vi "PI_GCS2_Sample_Application_2_Controllers.vi"() -> ()   [LabVIEW 2020]
doc: "This VI demonstrates how to initialize two PI GCS2 systems and how to query the help answers. \nThe diagram shows how to combine the driver VIs for these tasks. \n\nWarning: Before running this VI, modify the interface settings on the block diagram to reflect your configuration. The predefined settings provided with the VI probably do not match your system."
uses:
  Interface Settings.ctl
panel:
  out "Help string Sys. 2":string
  out "Identification Sys. 2":string
  out "Connected Axis System 2":string[](array[string])
  out "Help string Sys. 1":string
  in  "stop":bool
  in  "error in":errorcluster
  out "Running":bool caption="Configuration_Setup.vis running"
  out "error out":errorcluster
  out "Connected Axis System 1":string[](array[string])
  out "Identification Sys. 1":string
  # "This VI demonstrates how to initialize two PI GCS2 systems and how to query their help answer. \nThe diagram shows how to combine the driver VIs for these tasks. \n\nWarning: Before running this VI, modify the interface settings on the block diagram to reflect your configuration. The predefined \n                 settings provided with the VI probably do not match your system."
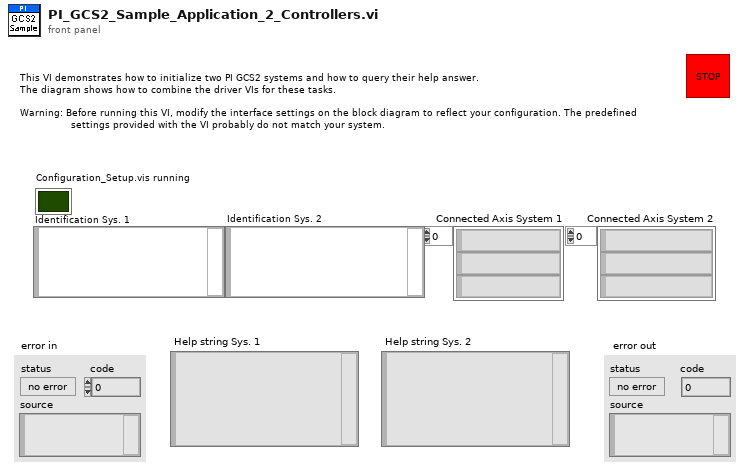
[diagram p1: front panel]
types:
  T1 = typedef "Interface Settings.ctl" = cluster{"Interface":u16, "Timeout":u32, "RS232 settings":cluster{"Portnumber":u8, "Baudrate":u16}, "TCP/IP settings":cluster{"Host address/name":string, "Port":i32, "Board":i32, "TCP/IP Search?":bool}, "USB settings":cluster{"S/N":string, "USB Search?":bool}, "DaisyChain settings":cluster{"Register DC":bool, "DaisyChain Search?":bool, "Device ID":i32}, "DLL for Device":u16}
  T2 = enum16{"Do not reference", "Reference switch", "Negative limit switch", "Positive limit switch"}[]
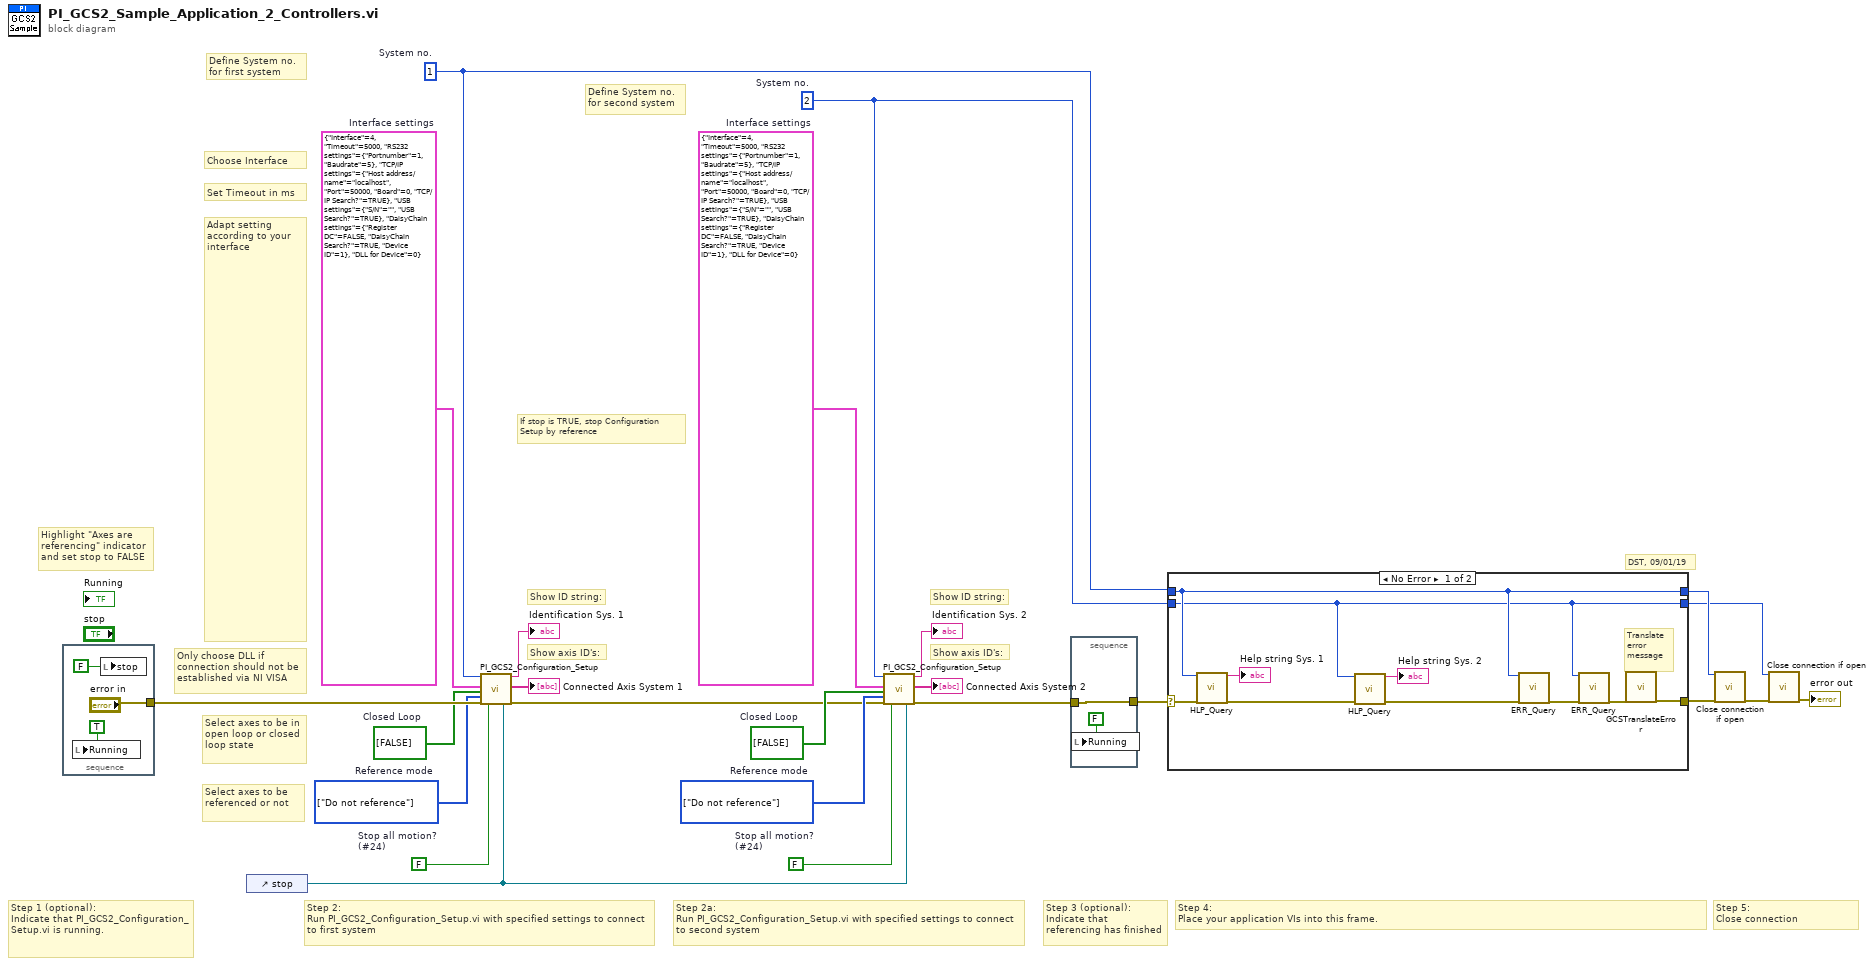
[diagram p0: block diagram]
diagram:
  w5 = T1 {"Interface"=4, "Timeout"=5000, "RS232 settings"={"Portnumber"=1, "Baudrate"=5}, "TCP/IP settings"={"Host address/name"="localhost", "Port"=50000, "Board"=0, "TCP/IP Search?"=TRUE}, "USB settings"={"S/N"="", "USB Search?"=TRUE}, "DaisyChain settings"={"Register DC"=FALSE, "DaisyChain Search?"=TRUE, "Device ID"=1}, "DLL for Device"=0}  # Interface settings
  w6 = T1 {"Interface"=4, "Timeout"=5000, "RS232 settings"={"Portnumber"=1, "Baudrate"=5}, "TCP/IP settings"={"Host address/name"="localhost", "Port"=50000, "Board"=0, "TCP/IP Search?"=TRUE}, "USB settings"={"S/N"="", "USB Search?"=TRUE}, "DaisyChain settings"={"Register DC"=FALSE, "DaisyChain Search?"=TRUE, "Device ID"=1}, "DLL for Device"=0}  # Interface settings
  w16 = FALSE  # Stop all motion? (#24)
  w15 = T2 [enum."Do not reference"] items=["Do not reference", "Reference switch", "Negative limit switch", "Positive limit switch"]  # Reference mode
  w14 = bool[] [FALSE]  # Closed Loop
  w4 = 2  # System no.
  w17 = FALSE  # Stop all motion? (#24)
  w18 = T2 [enum."Do not reference"] items=["Do not reference", "Reference switch", "Negative limit switch", "Positive limit switch"]  # Reference mode
  w19 = bool[] [FALSE]  # Closed Loop
  w2 = 1  # System no.
  # "Step 2a: \nRun PI_GCS2_Configuration_Setup.vi with specified settings to connect to second system"
  # "Define System no. for second system"
  # "Show axis ID's:"
  # "Show ID string:"
  # "Step 5: \nClose connection"
  # "Define System no.\nfor first system"
  # "Select axes to be referenced or not"
  # "Select axes to be in open loop or closed loop state"
  # "Adapt setting according to your interface"
  # "Set Timeout in ms"
  # "Choose Interface"
  # "Only choose DLL if connection should not be established via NI VISA"
  # "If stop is TRUE, stop Configuration\nSetup by reference"
  # "Step 4: \nPlace your application VIs into this frame."
  # "DST, 09/01/19"
  # "Step 3 (optional): \nIndicate that referencing has finished"
  # "Step 2: \nRun PI_GCS2_Configuration_Setup.vi with specified settings to connect to first system"
  # "Step 1 (optional): \nIndicate that PI_GCS2_Configuration_Setup.vi is running."
  # "Highlight \"Axes are\nreferencing\" indicator\nand set stop to FALSE"
  # "Show axis ID's:"
  # "Show ID string:"
  n1 = stacked-sequence {
    tunnel: ["error in"] -> w23
    frame #0 {
      n2 = local write "Running"(TRUE ("Running")) -> ()
      n3 = local write "stop"(FALSE ("stop")) -> ()
    }
  }
  n4 = control-ref of="stop"() -> (w10:refnum<vi>)
  n5 = call "PI_GCS2_Configuration_Setup.vi"("System no."=w2, "Interface settings"=w6, "Closed Loop"=w19, "Reference mode"=w18, "error in"=w23, "Stop all motion?"=w17, "Stop refnum"=w10) -> ("Identification"=→"Identification Sys. 1":string, "Conn. Axis"=→"Connected Axis System 1":string[], "error out"=w11:errorcluster)  [unwired: 1 in, 9 out]
  n6 = call "PI_GCS2_Configuration_Setup.vi"("System no."=w4, "Interface settings"=w5, "Closed Loop"=w14, "Reference mode"=w15, "error in"=w11, "Stop all motion?"=w16, "Stop refnum"=w10) -> ("Identification"=→"Identification Sys. 2":string, "Conn. Axis"=→"Connected Axis System 2":string[], "error out"=w9:errorcluster)  [unwired: 1 in, 9 out]
  n7 = stacked-sequence {
    tunnel: w9 -> [w28]
    tunnel: [w28] -> w22
    frame #0 {
      n8 = local write "Running"(FALSE ("Running")) -> ()
    }
  }
  n9 = case shown="No Error" w22 {
    selector: w22 -> [w37 w41]
    tunnel: [w38 w41] -> w8
    tunnel: w2 -> [w31 w40]
    tunnel: w4 -> [w30 w39]
    tunnel: [w31 w40] -> w3
    tunnel: [w30 w39] -> w1
    frame No Error {
      # "Translate\nerror \nmessage"
      n10 = call "HLP_Query.vi"("System no."=w31, "error in"=w37) -> ("Help string"=→"Help string Sys. 1":string, "error out"=w36:errorcluster)  [unwired: 16 out]
      n11 = call "HLP_Query.vi"("System no."=w30) -> ("Help string"=→"Help string Sys. 2":string)  [unwired: 1 in, 17 out]
      n12 = call "ERR_Query.vi"("System no."=w31, "error in"=w36) -> ("error out"=w33:errorcluster)  [unwired: 17 out]
      n13 = call "ERR_Query.vi"("System no."=w30, "error in"=w33) -> ("error out"=w32:errorcluster)  [unwired: 17 out]
      n14 = call "GCSTranslateError.vi"("error in"=w32) -> ("error out"=w38:errorcluster)  [unwired: 18 out]
    }
    frame Error {
      # "Error during initialization"
    }
  }
  n15 = call "Close connection if open.vi"("System no."=w3, "error in"=w8) -> ("error out"=w7:errorcluster)  [unwired: 1 in, 16 out]
  n16 = call "Close connection if open.vi"("System no."=w1, "error in"=w7) -> ("error out"=→"error out":errorcluster)  [unwired: 1 in, 16 out]
